vi "TestMods.vi"   [LabVIEW 2018]
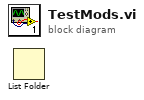
[diagram p0: block diagram]
diagram:
  n1 = List Folder() -> ()  [unwired: 4 in, 4 out]
